vi "Set Channel Values by Block Data Ref.vi"(8 "error in":errorcluster, 9 "Values in":dbl[](array[numeric]), 10 "Block Data Ref in":T1(array[cluster]) {"Data Reference" format="%.0x"}, 11 "NIVS Custom Device API in":refnum<class "NIVS Custom Device API.lvclass">) -> (0 "error out":errorcluster, 1 "Values out":dbl[](array[numeric]), 2 "Block Data Ref out":T1(array[cluster]) {"Data Reference" format="%.0x"}, 3 "NIVS Custom Device API out":refnum<class "NIVS Custom Device API.lvclass">)   [LabVIEW 2026, in "SystemMonitor Engine.lvlib" / "NIVS Custom Device API.lvclass"]
uses:
  NIVS Custom Device API.lvclass
  NIVS Custom Device API.lvclass/NIVS Custom Device API.ctl
  <vilib>/NI VeriStand/Custom Device API/Custom Device API.lvlib
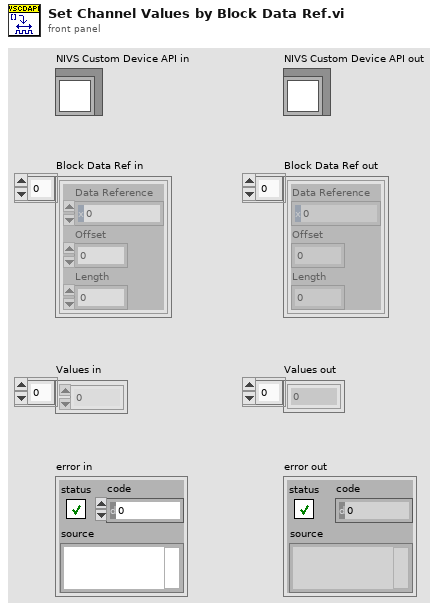
[diagram p1: front panel]
types:
  T1 = cluster{"Data Reference":i32, "Offset":u64, "Length":u64}[]
  T2 = typedef "Custom Device API.lvlib/Block Data Reference.ctl" = cluster{"Data Reference":T3, "Offset":u64, "Length":u64}
  T3 = typedef "Custom Device API.lvlib/Data Reference.ctl" = i32
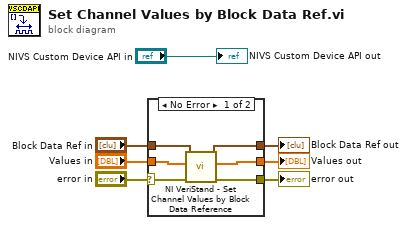
[diagram p0: block diagram]
diagram:
  n1 = case shown="No Error" "error in" {
    selector: "error in" -> [w13 w16]
    tunnel: [w12 w16] -> w5
    tunnel: [w11 w14] -> w2
    tunnel: [w10 w15] -> w3
    tunnel: "Block Data Ref in" -> [w9 w14]
    tunnel: "Values in" -> [w8 w15]
    frame No Error {
      n2 = call <vilib>:"NI VeriStand - Set Channel Values by Block Data Reference.vi"("error in (no error)"=w13, "Values Array in"=w8, "Block Data Ref"=w9) -> ("error out"=w12:errorcluster, "Values Array out"=w10:dbl[], "Block Data Ref dup"=w11:T2[])  [unwired: 6 in]
    }
    frame Error {
    }
  }
  "error out" <- w5
  "Values out" <- w3
  "Block Data Ref out" <- w2
  "NIVS Custom Device API out" <- "NIVS Custom Device API in"
